vi "3. Work with files.vi"() -> ()   [LabVIEW 2020]
panel:
  in  "file path (use dialog)":path
  out "Numeric 2":i32
  out "Numeric":i32
  in  "Array":string[][](array[string])=[["1", "2", "3"], ["4", "5", "6"], ["7", "8", "9"], ["10", "11", "12"]]
  # "Write the elements of the array one below the other in the file"
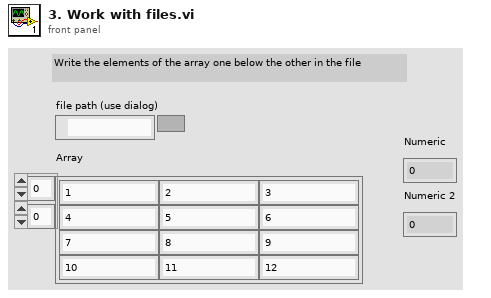
[diagram p1: front panel]
types:
  T1 = enum16{"open", "replace", "create", "open or create", "replace or create", "replace or create with confirmation"}
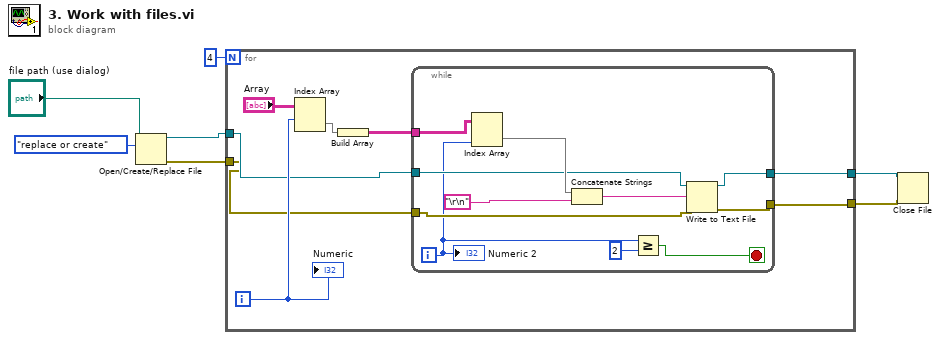
[diagram p0: block diagram]
diagram:
  n1 = Open/Create/Replace File(file path (use dialog)="file path (use dialog)", operation (0:open)=T1."replace or create") -> (refnum out=w6:refnum<file>, error out=w5:errorcluster)  [unwired: 4 in, 1 out]
  n2 = for {
    N: 4 -> [_]
    tunnel: w6 -> [w12]
    tunnel: w5 -> [w11]
    tunnel: [w9] -> w2
    tunnel: [w8] -> w1
    i -> [w14]
    n3 = Index Array(array="Array", index (row)=w14) -> (element=w13:string[])  [unwired: 1 in]
    n4 = Build Array(w13) -> (w10:string[][])
    n5 = while {
      tunnel: w12 -> [w22]
      tunnel: w11 -> [w21]
      tunnel: w10 -> [w26]
      tunnel: [w20] -> w8
      tunnel: [w19] -> w9
      i -> [w18]
      stop <- w16 stop-if-true
      n6 = Index Array(array=w26, index (col)=w18) -> (element=w23:string[])  [unwired: 1 in]
      n7 = Concatenate Strings(w23, "\r\n") -> (w25:string)
      n8 = Greater Or Equal?(x=w18, y=2) -> (x >= y?=w16:bool)
      n9 = Write to Text File(file (use dialog)=w22, text=w25, error in=w21) -> (refnum out=w20:refnum<file>, error out=w19:errorcluster)  [unwired: 1 in, 1 out]
      "Numeric 2" <- w18
    }
    "Numeric" <- w14
  }
  n10 = Close File(refnum=w1, error in=w2) -> ()  [unwired: 2 out]
